vi "WriteLogByRef.vi"(8 "ErrorIn":errorcluster, 9 "MessagesList":T1, 10 "InitString":string, 11 "RefStringIn":refnum<vi>) -> (0 "ErrorOut":errorcluster, 3 "RefStringOut":refnum<vi>)   [LabVIEW 2015]
uses:
  TypeDefs/StatusLogMessages.ctl
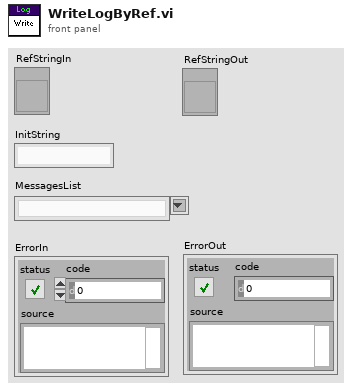
[diagram p1: front panel]
types:
  T1 = typedef "StatusLogMessages.ctl" = string
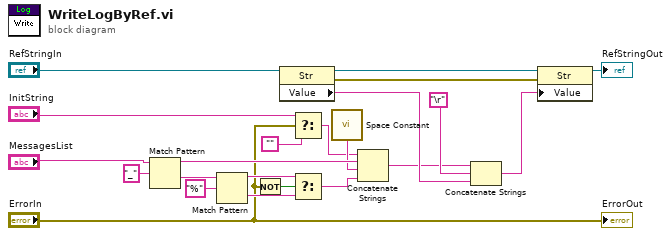
[diagram p0: block diagram]
diagram:
  n1 = Match Pattern(string="MessagesList", regular expression="_") -> (before substring=w14:T1, after substring=w13:T1)  [unwired: 1 in, 2 out]
  n2 = Match Pattern(string=w13, regular expression="%") -> (before substring=w10:T1, after substring=w9:T1)  [unwired: 1 in, 2 out]
  n3 = Not(x="ErrorIn") -> (.not. x?=w6:bool)
  n4 = property class="Str"(reference="RefStringIn") -> (reference out=w21:refnum<vi>, error out=w17:errorcluster, "Value"=w20:string)  [unwired: 1 in]
  n5 = Select(t="InitString", s="ErrorIn", f="") -> (s? t:f=w2:string)
  n6 = Select(t=w10, s=w6, f=w9) -> (s? t:f=w8:T1)
  n7 = call <vilib>:"Space Constant.vi"() -> ("String"=w11:string)
  n8 = Concatenate Strings(w2, w14, w11, w8) -> (w7:string)
  n9 = Concatenate Strings(w7, "\r", w20) -> (w18:string)
  n10 = property class="Str"(reference=w21, error in=w17, "Value"=w18) -> (reference out=→"RefStringOut":refnum<vi>)  [unwired: 1 out]
  "ErrorOut" <- "ErrorIn"
